vi "Poles_Placement.vi"(9 "Imaginary":dbl(knob)=-10.013861291935129 scale=0.0..-20.0 scale format="%#_4g", 10 "Real":dbl(knob)=-3.4076115316471642 scale=0.0..-22.0 scale format="%#_4g", 11 "State-Space Model":T1 {"Transport Delay" format="%.2f"; "D" format="%#.2g"; "C" format="%#.2g"; "B" format="%#.2g"; "A" format="%#.2g"; "properties"."Sampling Time" format="%#.6p"; "properties"."Output Delays" format="%.4f"; "properties"."Input Delays" format="%.4f"}) -> (1 "Gain":dbl[](array[numeric]), 2 "State Trajectory Graph":cluster{"time":dbl[], dbl[]}[](graph), 3 "Closed-Loop Step Response":cluster{"time":dbl[], dbl[]}[](graph), 4 "Actual Poles":cdb[](array[numeric])=[-4.9512521676495505+0.0i, -3.4076115316471447-10.013861291935113i, -3.4076115316471447+10.013861291935113i] format="%.2f", 5 "Desired Poles":cdb[](array[numeric])=[-4.951252167649562+0.0i, -3.4076115316471642-10.013861291935129i, -3.4076115316471642+10.013861291935129i] format="%.2f")   [LabVIEW 2011]
uses:
  <vilib>/addons/Control Design/_Model Construction/Model Typedefs.llb/CD State Space Model (MIMO).ctl
  <vilib>/addons/Control Design/_Model Construction/Model Typedefs.llb/CD General Elements.ctl
  <vilib>/addons/Control Design/_Model Construction/Data Typedefs.llb/CD Time Info.ctl
  <vilib>/Analysis/polynomials.llb/Sort Complex Numbers (obs).vi
  <vilib>/addons/Control Design/_State Feedback Control/State Feedback Control.llb/CD State Regulator.vi
  <vilib>/addons/Control Design/_Time Response Analysis/Time Response.llb/Time Response subVI/cd_Step Response (State-Space).vi
  <vilib>/Analysis/NI_AALPro.lvlib
  <vilib>/addons/Control Design/_Model Construction/NI_LinSys_Data Typedefs.lvlib
  <vilib>/addons/Control Design/_Time Response Analysis/NI_CD_Time Response.lvlib
  <vilib>/addons/Control Design/_State Feedback Control/NI_CD_State Feedback Control.lvlib
  <vilib>/addons/Control Design/_Model Construction/NI_LinSys_Model Typedefs.lvlib
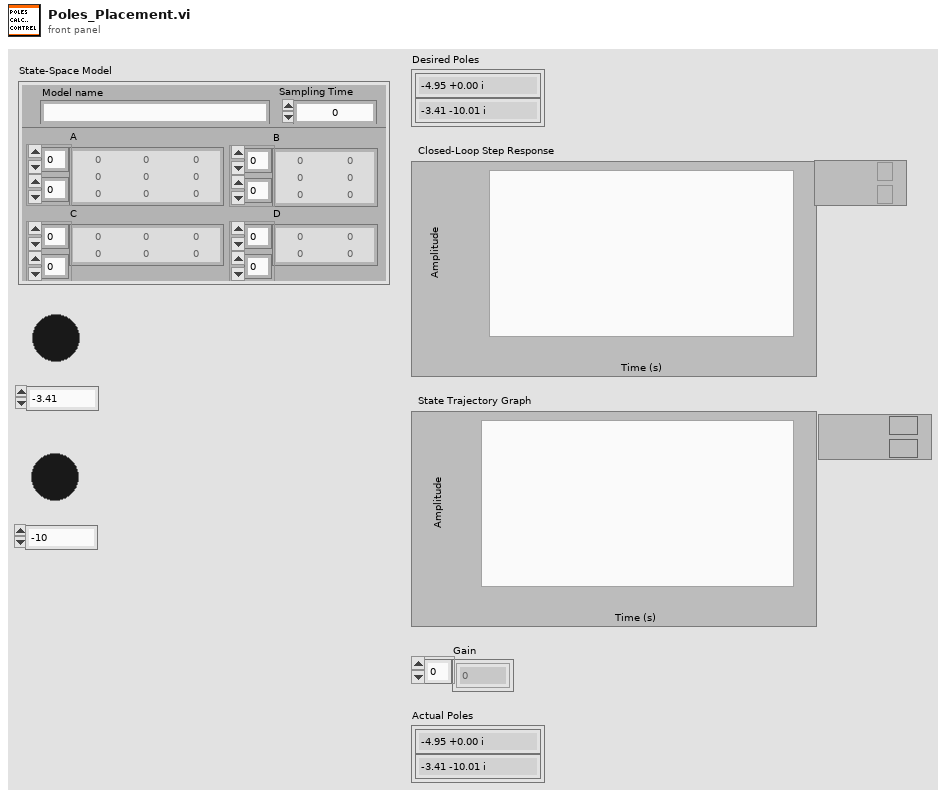
[diagram p1: front panel]
types:
  T1 = typedef "NI_LinSys_Model Typedefs.lvlib/CD State Space Model (MIMO).ctl" = cluster{"properties":T2, "A":dbl[][], "B":dbl[][], "C":dbl[][], "D":dbl[][], "StateNames":string[], "Transport Delay":dbl[][]}
  T2 = typedef "NI_LinSys_Model Typedefs.lvlib/CD General Elements.ctl" = cluster{"Model name":string, "Input names":string[], "Output names":string[], "Input Delays":dbl[], "Output Delays":dbl[], "Sampling Time":dbl, "Notes":string}
  T3 = typedef "NI_LinSys_Data Typedefs.lvlib/CD Time Info.ctl" = cluster{"t0":dbl, "dt":dbl, "tf":dbl}
  T4 = enum16{"System Included", "System Included with Noise", "Standalone"}
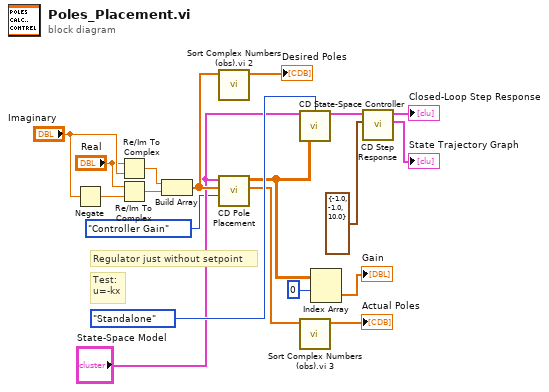
[diagram p0: block diagram]
diagram:
  # "Test:\nu=-kx"
  # "Regulator just without setpoint"
  n1 = Negate(x="Imaginary") -> (-x=w9:dbl)
  n2 = Re/Im To Complex(1:"Imaginary", 2:"Real") -> (0:w6:cdb)
  n3 = Re/Im To Complex(1:w9, 2:"Real") -> (0:w7:cdb)
  n4 = Build Array(w6, w7) -> (w3:cdb[])
  n5 = call "Sort Complex Numbers (obs).vi 2"("Complex Numbers"=w3) -> ("Sorted Complex Numbers"=→"Desired Poles":cdb[])  [unwired: 8 in, 2 out]
  n6 = call <vilib>:"CD Pole Placement.vi"("Gain Type"=enum16{"Controller Gain", "Observer Gain"}."Controller Gain" ("Type"), "Poles"=w3, "State-Space Model"="State-Space Model") -> ("Actual Poles"=w5:cdb[], "Gain"=w4:dbl[][])  [unwired: 6 in, 1 out]
  n7 = call-poly <vilib>:"CD State-Space Controller.vi"("State-Space Model"="State-Space Model", "Configuration"=T4."Standalone", "Controller Gain (K)"=w4) -> ("Controller Model"=w15:T1)  [unwired: 11 in, 1 out]
  n8 = call "Sort Complex Numbers (obs).vi 3"("Complex Numbers"=w5) -> ("Sorted Complex Numbers"=→"Actual Poles":cdb[])  [unwired: 8 in, 2 out]
  n9 = Index Array(array=w4, index (row)=0) -> (element=→"Gain":dbl[])  [unwired: 1 in]
  n10 = call-poly <vilib>:"CD Step Response.vi"("Time Range"=T3 {"t0"=-1.0, "dt"=-1.0, "tf"=10.0} ("Time Info"), "State-Space Model"=w15) -> ("State Trajectory Graph"=→"State Trajectory Graph":cluster{"time":dbl[], dbl[]}[], "Step Response Graph"=→"Closed-Loop Step Response":cluster{"time":dbl[], dbl[]}[])  [unwired: 6 in, 2 out]
